vi "添加数据.vi"(0 "数据输入":cluster{"扫描":T1[], "脉冲":T1[], "维持时间":T1[]}, 1 "新数据":cluster{"扫描":T1[], "脉冲":T1[], "维持时间":T1[]}) -> (2 "数据输出":cluster{"扫描":T1[], "脉冲":T1[], "维持时间":T1[]})   [LabVIEW 2021]
uses:
  3842a57f-4ea4-4c28-a00b-9af7a6fa7750.vi
  c24a25a2-3d8d-42df-a51b-b91af1b0c62b.vi
  a746ed54-61e7-4f5d-89cd-6729106411a7.vi
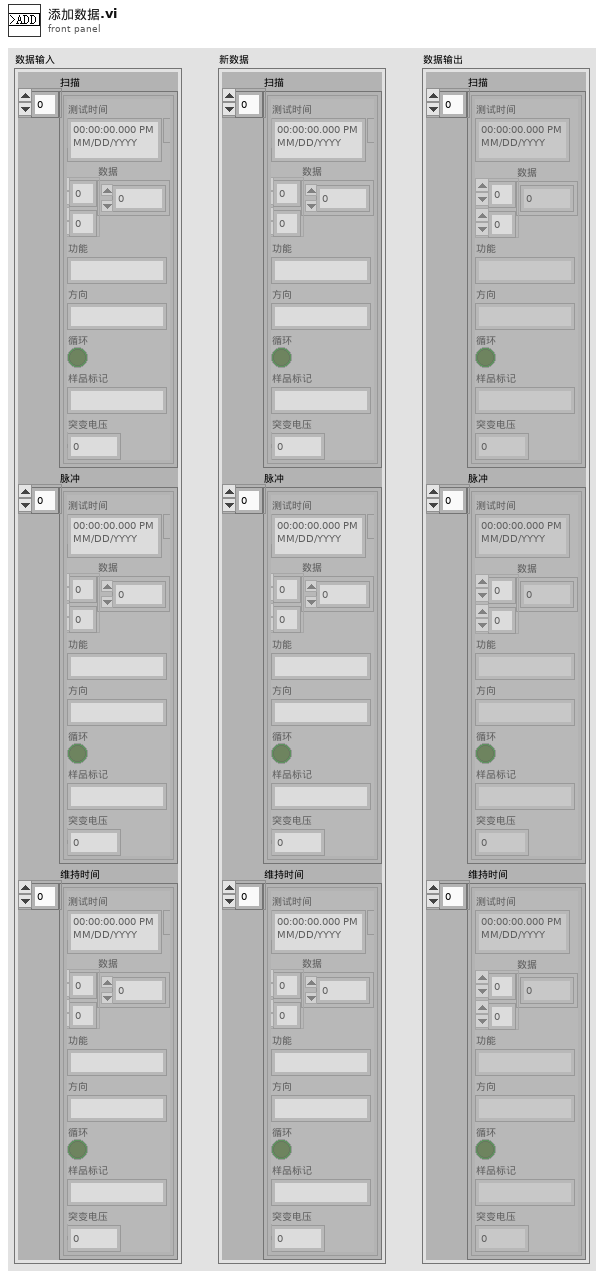
[diagram p1: front panel]
types:
  T1 = typedef "测试数据类型.ctl" = cluster{"测试时间":timestamp, "数据":dbl[][], "功能":string, "方向":string, "循环":bool, "样品标记":string, "突变电压":dbl}
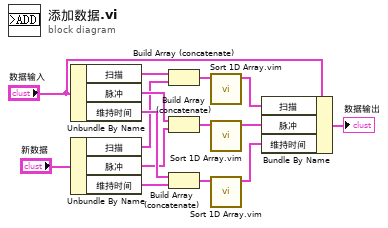
[diagram p0: block diagram]
diagram:
  n1 = Unbundle By Name("数据输入") -> ("扫描"=w2:T1[], "脉冲"=w4:T1[], "维持时间"=w6:T1[])
  n2 = Unbundle By Name("新数据") -> ("扫描"=w3:T1[], "脉冲"=w5:T1[], "维持时间"=w7:T1[])
  n3 = Build Array (concatenate)(w2, w3) -> (w8:T1[])
  n4 = Build Array (concatenate)(w4, w5) -> (w9:T1[])
  n5 = Build Array (concatenate)(w6, w7) -> (w10:T1[])
  n6 = call "Sort 1D Array.vim"("unsorted array"=w8) -> ("sorted array"=w12:T1[])  [unwired: 10 in]
  n7 = call "Sort 1D Array.vim"("unsorted array"=w9) -> ("sorted array"=w13:T1[])  [unwired: 10 in]
  n8 = call "Sort 1D Array.vim"("unsorted array"=w10) -> ("sorted array"=w14:T1[])  [unwired: 10 in]
  n9 = Bundle By Name(cluster="数据输入", "扫描"=w12, "脉冲"=w13, "维持时间"=w14) -> (→"数据输出":cluster{"扫描":T1[], "脉冲":T1[], "维持时间":T1[]})
